vi "Is var in acceptable range.vi"(1 "Variable":dbl, 2 "Acceptable plus minus":dbl) -> (0 "Acceptable":bool)   [LabVIEW 2019]
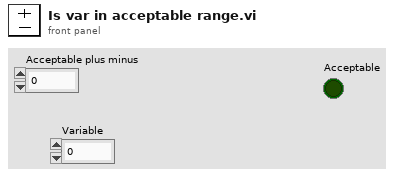
[diagram p1: front panel]
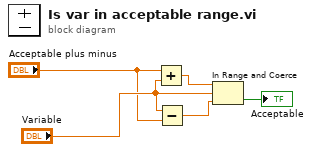
[diagram p0: block diagram]
diagram:
  n1 = Add(x="Acceptable plus minus", y="Variable") -> (x+y=w5:dbl)
  n2 = Subtract(x="Variable", y="Acceptable plus minus") -> (x-y=w4:dbl)
  n3 = In Range and Coerce(upper limit=w5, x="Variable", lower limit=w4) -> (In Range?=→"Acceptable":bool)  [unwired: 1 out]
